vi "AnalyseAndValidateTerminalNode.vi"(10 "Comparison VI":refnum<vi>, 11 "State":T1) -> (0 "Adapted VI":refnum<vi>, 1 "Invalid Terms":u8, 2 "Valid":bool, 3 "Terms":T2[](array[typedef]))   [LabVIEW 2012]
uses:
  <vilib>/XNodeSupport/XNodeTerm3.ctl
  <vilib>/XNodeSupport/XNodeString.ctl
  <vilib>/XNodeSupport/XNodeVariant.ctl
  <vilib>/XNodeSupport/XNodeRect32.ctl
  <vilib>/XNodeSupport/XNodeInt.ctl
  <vilib>/XNodeSupport/XNodeBool.ctl
  <vilib>/XNodeSupport/XNodeTermDirection.ctl
  State.ctl
  CThread.lvlib
  <vilib>/XNodeSupport/NI_XNodeSupport.lvlib
  CThread VI Terminal Node.xnode
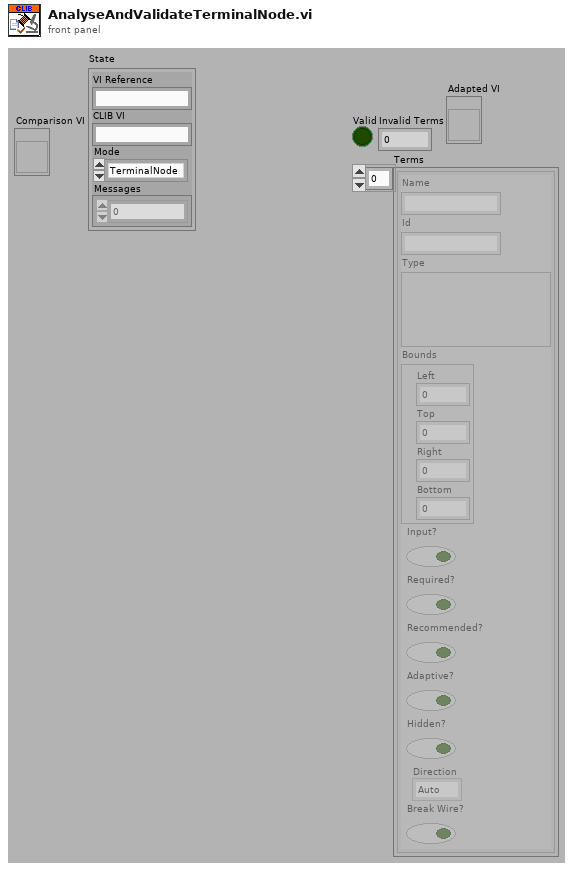
[diagram p1: front panel]
types:
  T1 = typedef "CThread.lvlib/CThread VI Terminal Node.xnode/State.ctl" = cluster{"VI Reference":string, "CLIB VI":string, "Mode":enum16{"TerminalNode", "AdaptorNode"}, "Messages":u8[]}
  T2 = typedef "NI_XNodeSupport.lvlib/XNodeTerm3.ctl" = cluster{"Name":T3, "Id":T3, "Type":T4, "Bounds":T5, "Input?":T7, "Required?":T7, "Recommended?":T7, "Adaptive?":T7, "Hidden?":T7, "Direction":T8, "Break Wire?":T7}
  T3 = typedef "NI_XNodeSupport.lvlib/XNodeString.ctl" = string
  T4 = typedef "NI_XNodeSupport.lvlib/XNodeVariant.ctl" = variant
  T5 = typedef "NI_XNodeSupport.lvlib/XNodeRect32.ctl" = cluster{"Left":T6, "Top":T6, "Right":T6, "Bottom":T6}
  T6 = typedef "NI_XNodeSupport.lvlib/XNodeInt.ctl" = i32
  T7 = typedef "NI_XNodeSupport.lvlib/XNodeBool.ctl" = bool
  T8 = typedef "NI_XNodeSupport.lvlib/XNodeTermDirection.ctl" = enum32{"Auto", "Up", "Down", "Left", "Right", "Center"}
  T9 = typedef "CRef.lvlib/Master Types.ctl" = enum8{"Null", "Boolean", "U8", "I8", "U16", "I16", "U32", "I32", "U64", "I64", "Single", "Double", "Extended", "CSG", "CDB", "CXT", "Boolean(Def)", "U8(Def)", "I8(Def)", "U16(Def)", "I16(Def)", "U32(Def)", "I32(Def)", "Reserved Def", "Reserved Def1", "Single(Def)", "Double(Def)", "Reserved Def2", "Reserved Def3", "Reserved Def4", "Reserved Def5", "Unsigned(Def)", "Signed(Def)", "Real(Def)", "Reserved Def6", "Numeric(Def)", "String"}
  T10 = typedef "LVRectTypeDef.ctl" = cluster{"Left":i16, "Top":i16, "Right":i16, "Bottom":i16}
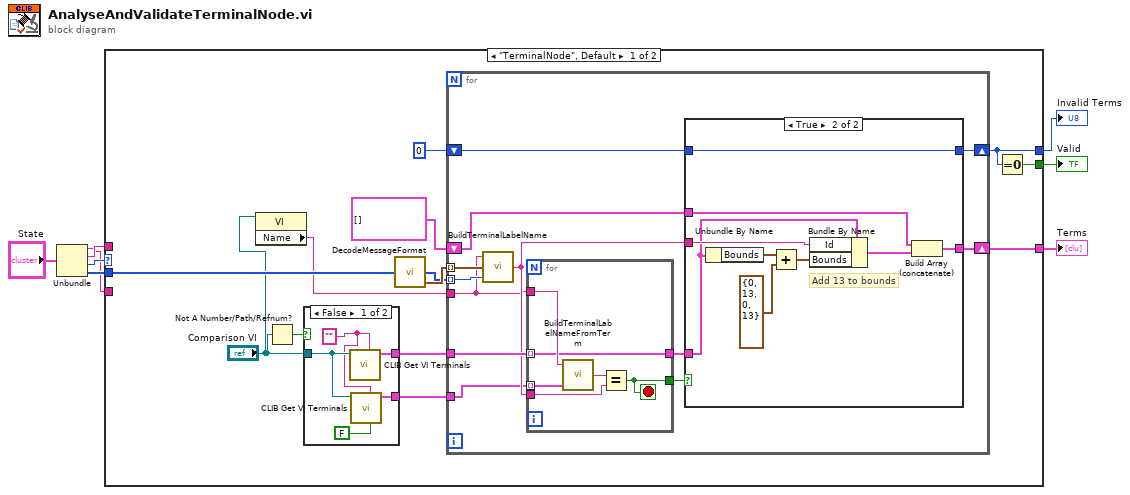
[diagram p0: block diagram]
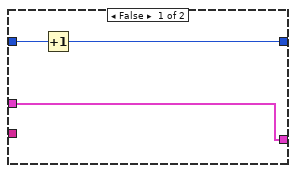
[diagram p3: hidden frame]
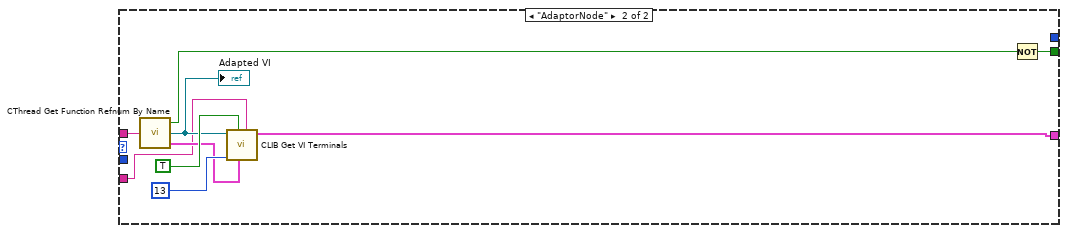
[diagram p4: hidden frame]
diagram:
  n1 = Unbundle("State") -> ("VI Reference"=w1:string, "CLIB VI"=w2:string, "Mode"=w4:enum16{"TerminalNode", "AdaptorNode"}, "Messages"=w3:u8[])
  n2 = case shown="\"TerminalNode\", Default" w4 {
    tunnel: w3 -> [w21 _]
    tunnel: w2 -> [_ w65]
    tunnel: w1 -> [_ w58]
    tunnel: [w13 w63] -> w8
    tunnel: [w14 _] -> w7
    tunnel: [w18 w57] -> w6
    frame "TerminalNode", Default {
      n3 = property class="VI"(reference="Comparison VI") -> ("Name"=w10:string)  [unwired: 1 in, 2 out]
      n4 = Not A Number/Path/Refnum?(number/path/refnum="Comparison VI") -> (NaN/Path/Refnum?=w15:bool)
      n5 = case shown="False" w15 {
        tunnel: "Comparison VI" -> [w25 _]
        tunnel: [w26 _] -> w17
        tunnel: [w24 _] -> w9
        frame False {
          w23 = "" ("VI-specific ID")
          n6 = call "CLIB Get VI Terminals.vi"("VI-specific ID"=w23, "reference"=w25) -> ("Terms"=w26:T2[])  [unwired: 8 in, 1 out]
          n7 = call "CLIB Get VI Terminals.vi"("Clip Edges (T)"=FALSE, "VI-specific ID"=w23, "reference"=w25) -> ("Terms"=w24:T2[])  [unwired: 7 in, 1 out]
        }
        frame True {
        }
      }
      n8 = call "DecodeMessageFormat.vi"("Messages"=w21) -> ("CRef Types"=w19:T9[], "Terminal Bounds[]"=w20:T10[])  [unwired: 2 in, 1 out]
      n9 = for {
        tunnel: w20 -> [w37] mode=indexing
        tunnel: w19 -> [w33] mode=indexing
        shift-right: [w32] -> w18
        shift-left: T2[] [] -> [w31]
        tunnel: w17 -> [w38]
        shift-right: [w30] -> w14
        shift-left: u8 0 -> [w29]
        tunnel: w10 -> [w28]
        tunnel: w9 -> [w27]
        n10 = call "BuildTerminalLabelName.vi"("CRef Type"=w33, "Bounds"=w37, "VI Name"=w28) -> ("Label Name"=w35:string)  [unwired: 1 in]
        n11 = for {
          tunnel: w38 -> [w53] mode=indexing
          tunnel: w28 -> [w56]
          tunnel: w35 -> [w52]
          tunnel: [w54] -> w36
          tunnel: [w53] -> w34
          tunnel: w27 -> [w51] mode=indexing
          stop <- w54 stop-if-true
          n12 = call "BuildTerminalLabelNameFromTerm.vi"("Term"=w51, "VI Name"=w56) -> ("Label Name"=w55:string)  [unwired: 2 in]
          n13 = Equal?(x=w55, y=w52) -> (x = y?=w54:bool)
        }
        n14 = case shown="True" w36 {
          tunnel: w35 -> [_ w47]
          tunnel: w34 -> [_ w45]
          tunnel: [w41 w50] -> w32
          tunnel: w31 -> [w41 w49]
          tunnel: w29 -> [w39 w48]
          tunnel: [w40 w48] -> w30
          frame False {
            n15 = Increment(x=w39) -> (x+1=w40:u8)
          }
          frame True {
            # "Add 13 to bounds"
            n16 = Unbundle By Name(w45) -> ("Bounds"=w44:T5)
            n17 = Add(x=w44, y=T5 {"Left"=0, "Top"=13, "Right"=0, "Bottom"=13}) -> (x+y=w43:T5)
            n18 = Bundle By Name(cluster=w45, "Id"=w47, "Bounds"=w43) -> (w46:T2)
            n19 = Build Array (concatenate)(w49, w46) -> (w50:T2[])
          }
        }
      }
      n20 = Equal To 0?(x=w14) -> (x = 0?=w13:bool)
    }
    frame "AdaptorNode" {
      n21 = call "CThread Get Function Refnum By Name.vi"("Name"=w65) -> ("Bounds"=w60:cluster{"Name":string, "Bounds":T5}[], "vi reference"=w59:refnum<vi>, "Failed"=w64:bool)
      "Adapted VI" <- w59
      n22 = call "CLIB Get VI Terminals.vi"("VI-specific ID"=w58, "Replacement Bounds"=w60, "RemoveRefTerminal?"=TRUE, "Y-Offset (0)"=i16 13 ("BoundsOffset-Y"), "reference"=w59) -> ("Terms"=w57:T2[])  [unwired: 5 in, 1 out]
      n23 = Not(x=w64) -> (.not. x?=w63:bool)
    }
  }
  "Valid" <- w8
  "Invalid Terms" <- w7
  "Terms" <- w6
